vi "Insert Data by Cluster Variant.vi"(4 "Drop Default Numeric? (F)":bool, 6 "Drop Default? (T)":bool=TRUE, 7 "data (VArray or Cluster)":variant, 8 "error in (no error)":errorcluster, 9 "columns":string[](array[string]), 10 "table":string, 11 "ADODB in":refnum<class "ADODB.lvclass">) -> (0 "error out":errorcluster, 3 "ADODB out":refnum<class "ADODB.lvclass">)   [LabVIEW 2020, in "ADODB.lvlib" / "ADODB.lvclass"]
uses:
  ADODB.lvclass
  ADODB.lvclass/ADODB.ctl
  DBMS Specific/DBMS Specific.lvclass
  <vilib>/addons/database/NI_Database_API.lvlib
  Database Reuse.lvlib
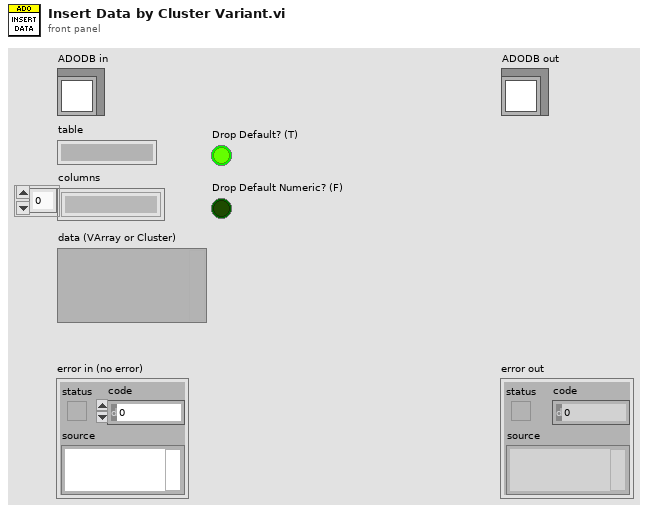
[diagram p1: front panel]
types:
  T1 = typedef "NI_Database_API.lvlib/Conn ObjectReference.ctl" = refnum<k1>
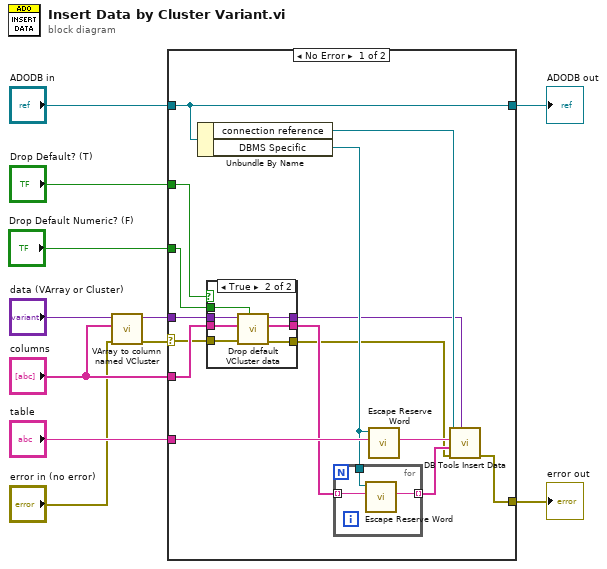
[diagram p0: block diagram]
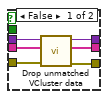
[diagram p2: hidden frame]
diagram:
  n1 = call "VArray to column named VCluster.vi"("error in (no error)"="error in (no error)", "columns"="columns", "data"="data (VArray or Cluster)") -> ("error out"=w2:errorcluster, "data (Cluster)"=w6:variant)  [unwired: 7 in]
  n2 = case shown="No Error" w2 {
    selector: w2 -> [w14 w44]
    tunnel: [w25 w44] -> w11
    tunnel: "ADODB in" -> [w24 w43]
    tunnel: [w24 w43] -> w9
    tunnel: "table" -> [w21 _]
    tunnel: "columns" -> [w17 _]
    tunnel: w6 -> [w19 _]
    tunnel: "Drop Default? (T)" -> [w15 _]
    tunnel: "Drop Default Numeric? (F)" -> [w12 _]
    frame No Error {
      n3 = Unbundle By Name(w24) -> ("connection reference"=w26:T1, "DBMS Specific"=w20:refnum<class "DBMS Specific.lvclass">)
      n4 = case shown="True" w15 {
        tunnel: w19 -> [w32 w39]
        tunnel: [w31 w38] -> w18
        tunnel: w17 -> [w29 w37]
        tunnel: [w28 w36] -> w16
        tunnel: w14 -> [w30 w35]
        tunnel: [w27 w34] -> w13
        tunnel: w12 -> [_ w33]
        frame False {
          n5 = call "Drop unmatched VCluster data.vi"("error in (no error)"=w30, "Columns"=w29, "VCluster in"=w32) -> ("error out"=w27:errorcluster, "VCluster Columns"=w28:string[], "VCluster out"=w31:variant)  [unwired: 6 in]
        }
        frame True {
          n6 = call "Drop default VCluster data.vi"("Drop default numeric? (F)"=w33, "error in (no error)"=w35, "Columns"=w37, "VCluster in"=w39) -> ("error out"=w34:errorcluster, "VCluster Columns"=w36:string[], "VCluster out"=w38:variant)  [unwired: 5 in]
        }
      }
      n7 = for {
        tunnel: w20 -> [w42]
        tunnel: w16 -> [w41] mode=indexing
        tunnel: [w40] -> w23 mode=indexing
        n8 = call-dynamic "Escape Reserve Word.vi"("Input Name"=w41, "DBMS Specific in"=w42) -> ("Escaped Name"=w40:string)  [unwired: 7 in, 2 out]
      }
      n9 = call-dynamic "Escape Reserve Word.vi"("Input Name"=w21, "DBMS Specific in"=w20) -> ("Escaped Name"=w22:string)  [unwired: 7 in, 2 out]
      n10 = call <vilib>:"DB Tools Insert Data.vi"("data"=w18, "error in (no error)"=w13, "columns"=w23, "table"=w22, "connection reference"=w26) -> ("error out"=w25:errorcluster)  [unwired: 5 in, 1 out]
    }
    frame Error {
    }
  }
  "error out" <- w11
  "ADODB out" <- w9
